vi "dau_dis.vi"() -> ()   [LabVIEW 2009]
uses:
  <userlib>/AotfLibrary/AotfLibrary.lvlib
panel:
  out "concatenated string 7":string
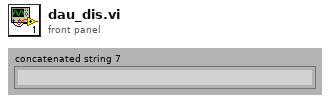
[diagram p1: front panel]
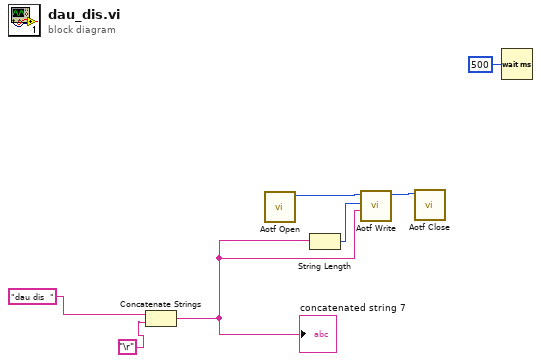
[diagram p0: block diagram]
diagram:
  n1 = Concatenate Strings("dau dis  " ("string"), "\r") -> (w3:string)
  "concatenated string 7" <- w3
  n2 = call <userlib>:"Aotf Open.vi"() -> ("function return"=w6:u32)  [unwired: 11 in]
  n3 = String Length(string=w3) -> (length=w5:i32)
  n4 = call <userlib>:"Aotf Write.vi"("pData"=w3, "uiLength"=w5, "hAotfController"=w6) -> ("hAotfController out"=w7:u32)  [unwired: 7 in, 1 out]
  n5 = call <userlib>:"Aotf Close.vi"("hAotfController"=w7) -> ()  [unwired: 9 in, 2 out]
  n6 = Wait (ms)(milliseconds to wait=u32 500) -> ()  [unwired: 1 out]
